vi "Command Test.vi"   [LabVIEW 2017]
uses:
  AT901 API/TypeDefinitions/ES_MeasMode.ctl
types:
  T1 = typedef "ES_MeasMode.ctl" = enum32{"ES_MM_Stationary", "ES_MM_ContinuousTime", "ES_MM_ContinuousDistance", "ES_MM_Grid", "ES_MM_SphrereCenter", "ES_MM_CircleCenter", "ES_MM_6DStationary", "ES_MM_6DContinuousTime", "ES_MM_6DContinuousDistance", "ES_MM_6DGrid", "ES_MM_6DSphrereCenter", "ES_MM6DCircleCenter"}
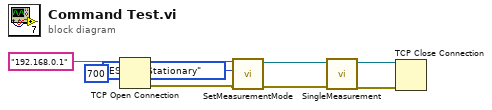
[diagram p0: block diagram]
diagram:
  n1 = TCP Open Connection(address="192.168.0.1", remote port or service name=u16 700) -> (connection ID=w5:refnum<k5>, error out=w4:errorcluster)  [unwired: 3 in]
  n2 = call "SetMeasurementMode.vi"("error in (no error)"=w4, "ES_MeasMode"=ES_MeasMode."ES_MM_Stationary", "TCP Network Connection in"=w5) -> ("error out"=w3:errorcluster, "TCP Network Connection out"=w2:refnum<k5>)  [unwired: 5 in, 2 out]
  n3 = call "SingleMeasurement.vi"("error in (no error)"=w3, "TCP Network Connection in"=w2) -> ("error out"=w6:errorcluster, "TCP Network Connection out"=w7:refnum<k5>)  [unwired: 5 in, 3 out]
  n4 = TCP Close Connection(connection ID=w7, error in (no error)=w6) -> ()  [unwired: 1 in, 2 out]
